vi "text column to array.vi"() -> ()   [LabVIEW 2020]
panel:
  out "array":string[](array[string])
  in  "column of data":string
  # "when copying from bullet points list, hold down alt button while copying from document\nto remove the buttets."
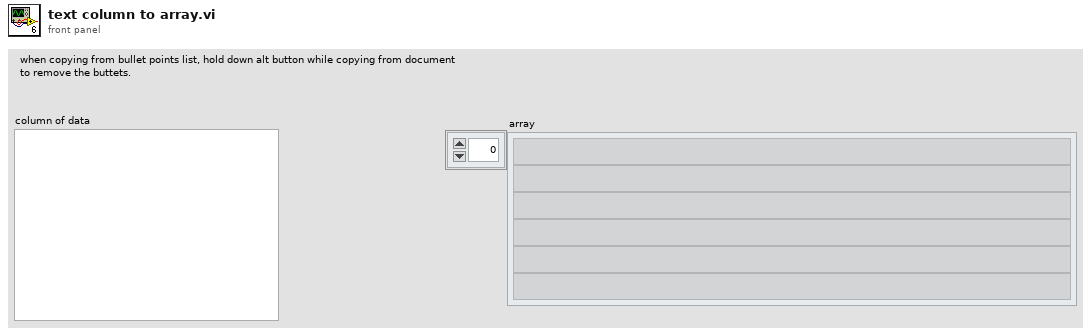
[diagram p1: front panel]
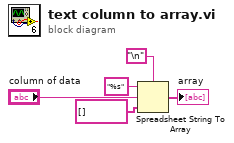
[diagram p0: block diagram]
diagram:
  n1 = Spreadsheet String To Array(delimiter (Tab)="\n", format string="%s", spreadsheet string="column of data", array type (2D Dbl)=string[] []) -> (array=→"array":string[])
